vi "GE 5565PIORC.VISA.Move In (DBL).vi"(5 "byte order (big-endian)":T1(ring), 7 "address space":T2=1 items=["VXI/VME A16"=1, "VXI/VME A24"=2, "VXI/VME A32"=3, "VXI/VME A64"=4, "PXI Memory Allocations"=9, "PXI Configuration"=10, "PXI BAR0"=11, "PXI BAR1"=12, "PXI BAR2"=13, "PXI BAR3"=14, "PXI BAR4"=15, "PXI BAR5"=16], 8 "error in (no error)":errorcluster, 9 "count":u32, 10 "offset":u32, 11 "VISA resource name":refnum<visa-resource-name>) -> (0 "error out":errorcluster, 1 "data out":dbl[](array[numeric]), 3 "VISA resource name out":refnum<visa-resource-name>)   [LabVIEW 2016, in "GE 5565PIORC.lvclass"]
uses:
  GE 5565PIORC.lvclass
  <vilib>/Instr/_visa.llb/VISA Register Access Address Space.ctl
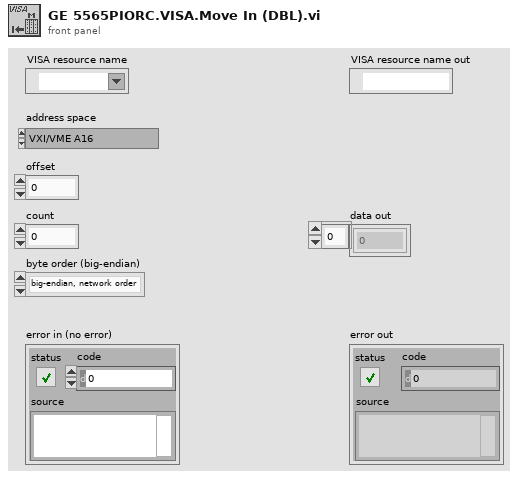
[diagram p1: front panel]
types:
  T1 = enum16{"big-endian, network order", "native, host order", "little-endian"}
  T2 = typedef "VISA Register Access Address Space.ctl" = u16
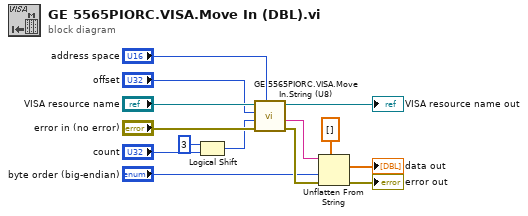
[diagram p0: block diagram]
diagram:
  n1 = Logical Shift(y=i16 3, x="count") -> (x << y=w7:u32)
  n2 = call "GE 5565PIORC.VISA.Move In.String (U8).vi"("address space"="address space", "error in (no error)"="error in (no error)", "count"=w7, "offset"="offset", "GE 5565PIORC in"="VISA resource name") -> ("error out"=w6:errorcluster, "data out"=w4:string, "GE 5565PIORC out"=→"VISA resource name out":refnum<class "GE 5565PIORC.lvclass">)  [unwired: 4 in]
  n3 = Unflatten From String(type=dbl[] [], binary string=w4, byte order (0:big-endian, network order)="byte order (big-endian)", error in (no error)=w6) -> (value=→"data out":dbl[], error out=→"error out":errorcluster)  [unwired: 1 in, 1 out]
